vi "Get Name.vi"(8 "error in (no error)":errorcluster, 11 "SMO":refnum<class "SMO.lvclass">) -> (0 "error out":errorcluster, 2 "Name":string, 3 "SMO out":refnum<class "SMO.lvclass">)   [LabVIEW 2013, in "SMO.lvclass"]
uses:
  SMO.lvclass
  Support/Attribute.Identity/Attribute.Identity.lvclass
  Support/Attribute.Identity/Attribute.Identity.lvclass/Attribute.Identity.ctl
  Support/Attribute/Attribute.lvclass
panel:
  # "For instructions on how to use the JKI State Machine Objects, examples and video tutorials, visit:\nhttp://jki.net/state-machine-objects/\n\nJKI State Machine Objects™\nhttp://jki.net/state-machine-objects/\nCopyright (C) 2005-2015, JKI <info@jki.net>\nALL RIGHTS RESERVED"
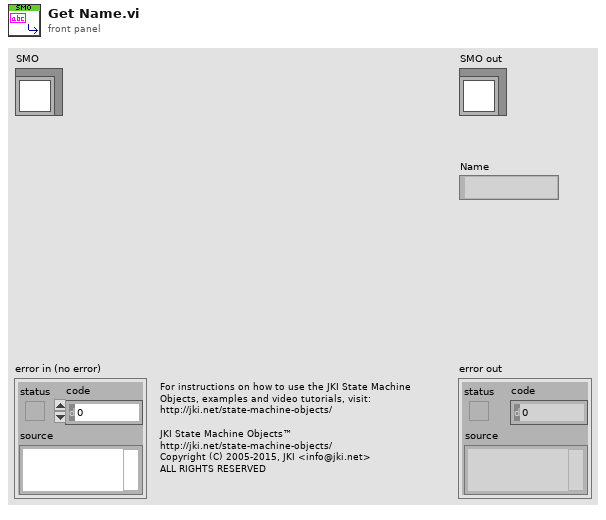
[diagram p1: front panel]
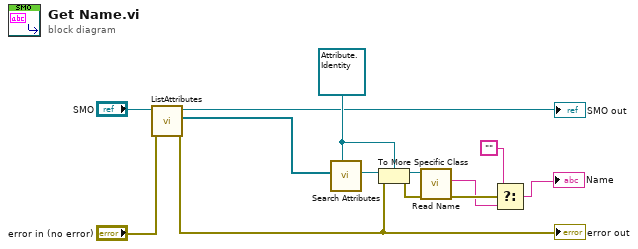
[diagram p0: block diagram]
diagram:
  w12 = refnum<class "Attribute.Identity.lvclass"> refnum ("Attribute.Identity.lvclass")
  n1 = call "ListAttributes.vi"("error in (no error)"="error in (no error)", "SMO in"="SMO") -> ("error out"=w2:errorcluster, "[Attributes]"=w3:refnum<class "Attribute.lvclass">[], "SMO out"=→"SMO out":refnum<class "SMO.lvclass">)  [unwired: 7 in]
  "error out" <- w2
  n2 = call "Search Attributes.vi"("Attribute type"=w12, "[Attributes]"=w3) -> ("Attribute out"=w13:refnum<class "Attribute.lvclass">)  [unwired: 8 in, 1 out]
  n3 = To More Specific Class(target class=w12, reference=w13, error in=w2) -> (specific class reference=w11:refnum<class "Attribute.Identity.lvclass">, error out=w10:errorcluster)
  n4 = call "Read Name.vi"("error in (no error)"=w10, "Attribute.Identity in"=w11) -> ("error out"=w9:errorcluster, "Name"=w8:string)  [unwired: 7 in, 1 out]
  n5 = Select(t="", s=w9, f=w8) -> (s? t:f=→"Name":string)
